vi "ServiceModeTest5.vi"(7 "Erd_ParametricVersion ERD #":T1={"ERD Number"=59, "Data Type"=enum."string"} {"ERD Number" format="%.0x"}, 8 "Error In":errorcluster, 9 "UI GEA Inputs":T5={"Source"=228, "Destination"=37} {"Destination" format="%.0x"; "Source" format="%.0x"}, 10 "MC GEA Inputs":T5={"Source"=228, "Destination"=36} {"Destination" format="%.0x"; "Source" format="%.0x"}, 11 "GEA2 Reference In":refnum<k24>) -> (0 "Error Out":errorcluster, 1 "Report Text":string, 2 "Pass/Fail?":bool, 3 "GEA2 Reference Out":refnum<k24>)   [LabVIEW 2016]
uses:
  Q:/Common/DLLs/GEA3/GeaCommunication.dll
  Common/DLLs/GEA3/GeaCommunication.dll
  Common/LabVIEW GEA2 Toolkit/LabVIEW_GEA2_Toolkit.lvlibp/type defs/Source_Destination.ctl
  Centauro Washer/Product Testcode/Centauro/Valew Common/type defs/LED Status OOB.ctl
  Common/LabVIEW GEA2 Toolkit/LabVIEW_GEA2_Toolkit.lvlibp/type defs/ERD Read Data In.ctl
  Common/LabVIEW GEA2 Toolkit/LabVIEW_GEA2_Toolkit.lvlibp/type defs/Data Type.ctl
  Common/Type Defs/JL_Buttons.ctl
  Common/LabVIEW GEA2 Toolkit/LabVIEW_GEA2_Toolkit.lvlibp
panel:
  in  "LED Status Cluster":T4
  in  "Board Index":i32
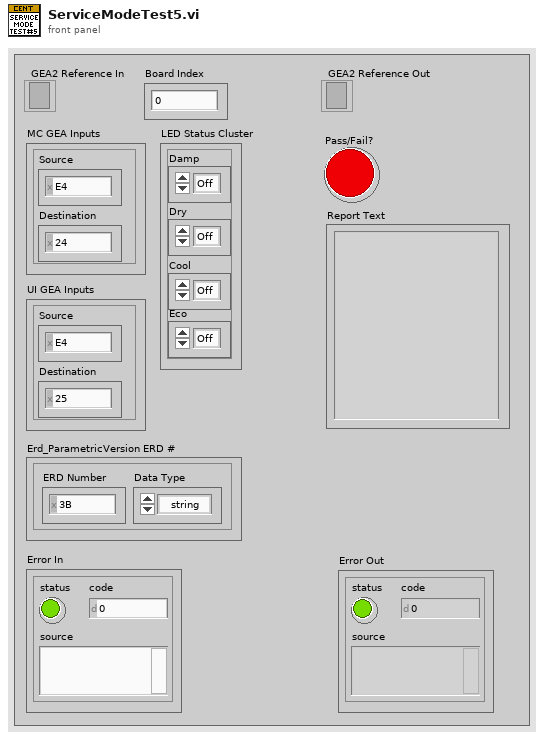
[diagram p1: front panel]
types:
  T1 = typedef "LabVIEW_GEA2_Toolkit.lvlibp/ERD Read Data In.ctl" = cluster{"ERD Number":u16, "Data Type":T2}
  T2 = typedef "LabVIEW_GEA2_Toolkit.lvlibp/Data Type.ctl" = enum16{"string", "boolean", "uint8_t", "uint16_t", "uint32_t", "uint64_t", "int8_t", "int16_t", "int32_t", "int64_t"}
  T3 = typedef "LED Status OOB.ctl" = enum32{"Off", "On", "Blink"}
  T4 = cluster{"Damp":T3, "Dry":T3, "Cool":T3, "Eco":T3}
  T5 = typedef "LabVIEW_GEA2_Toolkit.lvlibp/Source_Destination.ctl" = cluster{"Source":u8, "Destination":u8}
  T6 = typedef "LabVIEW_GEA2_Toolkit.lvlibp/ERD Read Data Out.ctl" = cluster{"ERD Number":u16, "Data":string}
  T7 = typedef "JL_Buttons.ctl" = enum16{"Power", "Start / Pause ", "Temp Option ", "Dryness Level", "Time Option", "Time Increment ", "Time Decrement ", "MyCycle", "eDry ", "Delay", "Extended Tumble", "Control Lock", "Volume/Signal", "Damp Alert / Drum Light", "Unused", "(SW213)", "(SW322)", "Clear / Reset"}
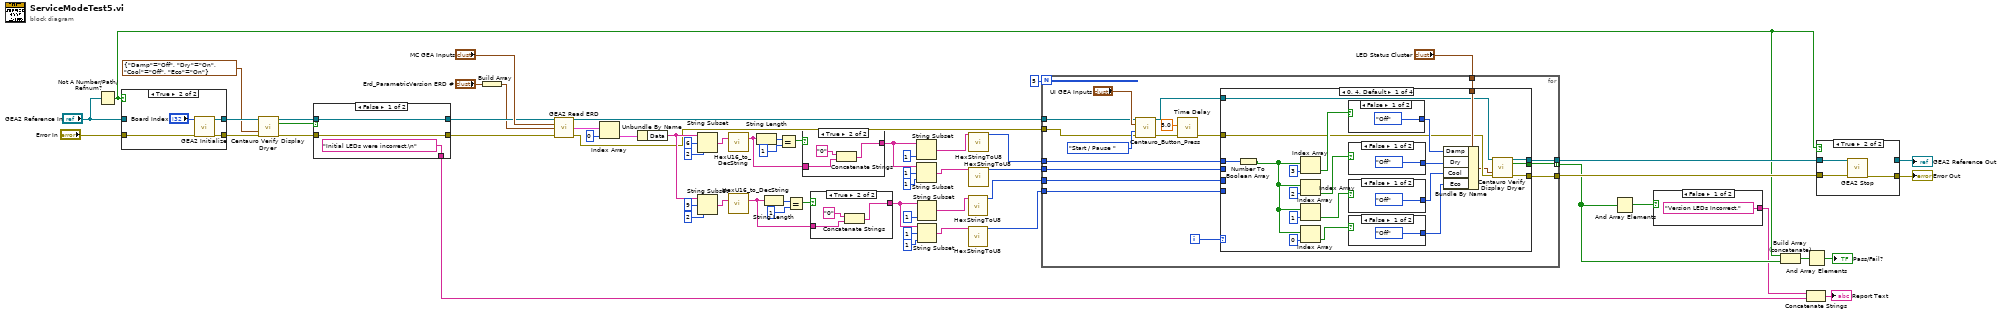
[diagram p0: block diagram]
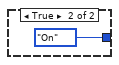
[diagram p5: hidden frame]
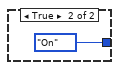
[diagram p6: hidden frame]
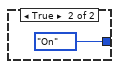
[diagram p7: hidden frame]
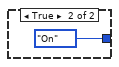
[diagram p8: hidden frame]
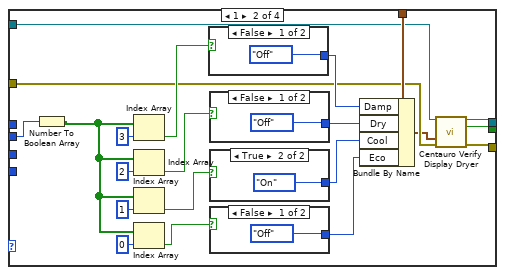
[diagram p9: hidden frame]
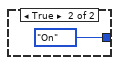
[diagram p10: hidden frame]
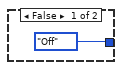
[diagram p11: hidden frame]
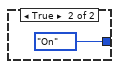
[diagram p12: hidden frame]
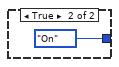
[diagram p13: hidden frame]
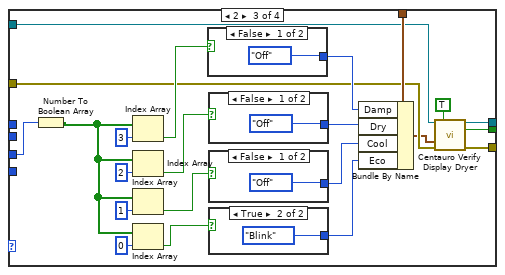
[diagram p14: hidden frame]
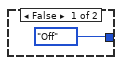
[diagram p15: hidden frame]
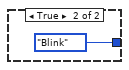
[diagram p16: hidden frame]
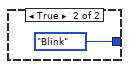
[diagram p17: hidden frame]
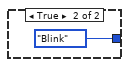
[diagram p18: hidden frame]
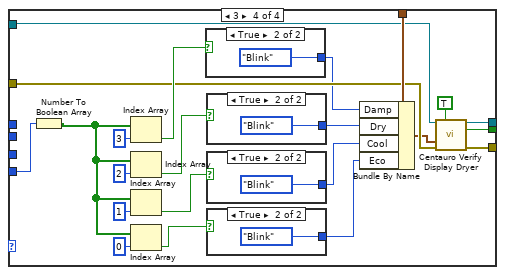
[diagram p19: hidden frame]
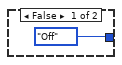
[diagram p20: hidden frame]
diagram:
  n1 = Not A Number/Path/Refnum?(number/path/refnum="GEA2 Reference In") -> (NaN/Path/Refnum?=w31:bool)
  n2 = case shown="True" w31 {
    tunnel: [w64 w69] -> w60
    tunnel: "Error In" -> [w64 w68]
    tunnel: [w65 w67] -> w61
    tunnel: "GEA2 Reference In" -> [w65 _]
    frame False {
    }
    frame True {
      n3 = call "GEA2 Initialize.vi"("Board Index"="Board Index", "error in"=w68) -> ("GEA2 Reference Out"=w67:refnum<k24>, "error out"=w69:errorcluster)  [unwired: 11 in, 1 out]
    }
  }
  n4 = call "Centauro Verify Display Dryer.vi"("GEA2 Reference In"=w61, "Expected LED Status"=T4 {"Damp"=enum."Off", "Dry"=enum."On", "Cool"=enum."Off", "Eco"=enum."On"}, "Error In"=w60) -> ("GEA2 Reference Out"=w59:refnum<k24>, "Pass/Fail?"=w53:bool, "Error Out"=w58:errorcluster)  [unwired: 7 in, 3 out]
  n5 = case shown="False" w53 {
    tunnel: w59 -> [w72 w74]
    tunnel: [w72 w74] -> w43
    tunnel: [w71 w73] -> w42
    tunnel: w58 -> [w71 w73]
    tunnel: ["Initial LEDs were incorrect.\n" _] -> w52
    frame False {
    }
    frame True {
    }
  }
  n6 = Build Array("Erd_ParametricVersion ERD #") -> (w2:T1[])
  n7 = call "GEA2 Read ERD.vi"("GEA2 Reference In"=w43, "GEA Inputs"="MC GEA Inputs", "Read ERD List"=w2, "Error In"=w42) -> ("GEA2 Reference Out"=w41:refnum<k24>, "ERD Data Out"=w56:T6[], "Error Out"=w40:errorcluster)  [unwired: 8 in, 1 out]
  n8 = Index Array(array=w56, index=0) -> (element=w54:T6)
  n9 = Unbundle By Name(w54) -> ("Data"=w45:string)
  n10 = String Subset(string=w45, offset (0)=6, length (rest)=2 ("length (rest)")) -> (substring=w25:string)
  n11 = String Subset(string=w45, offset (0)=9, length (rest)=2 ("length (rest)")) -> (substring=w24:string)
  n12 = call "HexU16_to_DecString.vi"("String"=w25) -> ("decimal integer string"=w20:string)  [unwired: 13 in, 1 out]
  n13 = call "HexU16_to_DecString.vi"("String"=w24) -> ("decimal integer string"=w16:string)  [unwired: 13 in, 1 out]
  n14 = String Length(string=w20) -> (length=w23:i32)
  n15 = String Length(string=w16) -> (length=w19:i32)
  n16 = Equal?(x=w23, y=1) -> (x = y?=w21:bool)
  n17 = Equal?(x=w19, y=1) -> (x = y?=w17:bool)
  n18 = case shown="True" w21 {
    tunnel: w20 -> [w75 w77]
    tunnel: [w75 w76] -> w14
    frame False {
    }
    frame True {
      n19 = Concatenate Strings("0" ("string"), w77) -> (w76:string)
    }
  }
  n20 = case shown="True" w17 {
    tunnel: w16 -> [w79 w81]
    tunnel: [w79 w80] -> w6
    frame False {
    }
    frame True {
      n21 = Concatenate Strings("0" ("string"), w81) -> (w80:string)
    }
  }
  n22 = String Subset(string=w14, length (rest)=1 ("length (rest)")) -> (substring=w11:string)  [unwired: 1 in]
  n23 = String Subset(string=w14, offset (0)=1, length (rest)=1 ("length (rest)")) -> (substring=w10:string)
  n24 = String Subset(string=w6, length (rest)=1 ("length (rest)")) -> (substring=w5:string)  [unwired: 1 in]
  n25 = String Subset(string=w6, offset (0)=1, length (rest)=1 ("length (rest)")) -> (substring=w4:string)
  n26 = call "HexStringToU8.vi"("Input String"=w5) -> ("Number Out"=w37:u8)  [unwired: 14 in]
  n27 = call "HexStringToU8.vi"("Input String"=w4) -> ("Number Out"=w36:u8)  [unwired: 14 in]
  n28 = call "HexStringToU8.vi"("Input String"=w11) -> ("Number Out"=w39:u8)  [unwired: 14 in]
  n29 = call "HexStringToU8.vi"("Input String"=w10) -> ("Number Out"=w38:u8)  [unwired: 14 in]
  n30 = for {
    N: 5 -> [_]
    tunnel: w41 -> [w96]
    tunnel: w40 -> [w95]
    tunnel: w39 -> [w94]
    tunnel: w38 -> [w93]
    tunnel: w37 -> [w92]
    tunnel: w36 -> [w91]
    tunnel: "LED Status Cluster" -> [w90]
    tunnel: [w88] -> w32 mode=indexing
    tunnel: [w87] -> w34
    tunnel: [w86] -> w33
    i -> [w99]
    n31 = call "Centauro_Button_Press.vi"("GEA2 Reference In"=w96, "GEA Inputs"="UI GEA Inputs", "Button"=JL_Buttons."Start / Pause ", "Error In"=w95) -> ("GEA2 Reference Out"=w89:refnum<k24>, "Error Out"=w84:errorcluster)  [unwired: 10 in]
    n32 = call "Time Delay"("error in (no error)"=w84, "Delay Time (s)"=5.0) -> ("error out"=w83:errorcluster)  [unwired: 9 in]
    n33 = case shown="0, 4, Default" w99 {
      tunnel: w94 -> [w120 _ _ _]
      tunnel: w93 -> [_ w140 _ _]
      tunnel: w92 -> [_ _ w170 _]
      tunnel: w91 -> [_ _ _ w200]
      tunnel: w90 -> [w110 w139 w169 w199]
      tunnel: w89 -> [w105 w134 w164 w198]
      tunnel: w83 -> [w104 w133 w163 w197]
      tunnel: [w103 w132 w162 w196] -> w88
      tunnel: [w102 w131 w161 w195] -> w87
      tunnel: [w101 w130 w160 w194] -> w86
      frame 0, 4, Default {
        n34 = Number To Boolean Array(number=w120) -> (Boolean array=w115:bool[])
        n35 = Index Array(array=w115, index=3) -> (element=w114:bool)
        n36 = Index Array(array=w115, index=2) -> (element=w113:bool)
        n37 = Index Array(array=w115, index=1) -> (element=w112:bool)
        n38 = Index Array(array=w115, index=0) -> (element=w111:bool)
        n39 = case shown="False" w114 {
          tunnel: [LED_Status_OOB."Off" ("Damp") LED_Status_OOB."On" ("Damp")] -> w109
          frame False {
          }
          frame True {
          }
        }
        n40 = case shown="False" w113 {
          tunnel: [LED_Status_OOB."Off" ("Damp") LED_Status_OOB."On" ("Damp")] -> w108
          frame False {
          }
          frame True {
          }
        }
        n41 = case shown="False" w112 {
          tunnel: [LED_Status_OOB."Off" ("Damp") LED_Status_OOB."On" ("Damp")] -> w107
          frame False {
          }
          frame True {
          }
        }
        n42 = case shown="False" w111 {
          tunnel: [LED_Status_OOB."Off" ("Damp") LED_Status_OOB."On" ("Damp")] -> w106
          frame False {
          }
          frame True {
          }
        }
        n43 = Bundle By Name(cluster=w110, "Damp"=w109, "Dry"=w108, "Cool"=w107, "Eco"=w106) -> (w100:T4)
        n44 = call "Centauro Verify Display Dryer.vi"("GEA2 Reference In"=w105, "Expected LED Status"=w100, "Error In"=w104) -> ("GEA2 Reference Out"=w102:refnum<k24>, "Pass/Fail?"=w103:bool, "Error Out"=w101:errorcluster)  [unwired: 7 in, 3 out]
      }
      frame 1 {
        n45 = Number To Boolean Array(number=w140) -> (Boolean array=w145:bool[])
        n46 = Index Array(array=w145, index=3) -> (element=w144:bool)
        n47 = Index Array(array=w145, index=2) -> (element=w143:bool)
        n48 = Index Array(array=w145, index=1) -> (element=w142:bool)
        n49 = Index Array(array=w145, index=0) -> (element=w141:bool)
        n50 = case shown="False" w144 {
          tunnel: [LED_Status_OOB."Off" ("Damp") LED_Status_OOB."On" ("Damp")] -> w138
          frame False {
          }
          frame True {
          }
        }
        n51 = case shown="False" w143 {
          tunnel: [LED_Status_OOB."Off" ("Damp") LED_Status_OOB."On" ("Damp")] -> w137
          frame False {
          }
          frame True {
          }
        }
        n52 = case shown="True" w142 {
          tunnel: [LED_Status_OOB."Off" ("Damp") LED_Status_OOB."On" ("Damp")] -> w136
          frame False {
          }
          frame True {
          }
        }
        n53 = case shown="False" w141 {
          tunnel: [LED_Status_OOB."Off" ("Damp") LED_Status_OOB."On" ("Damp")] -> w135
          frame False {
          }
          frame True {
          }
        }
        n54 = Bundle By Name(cluster=w139, "Damp"=w138, "Dry"=w137, "Cool"=w136, "Eco"=w135) -> (w129:T4)
        n55 = call "Centauro Verify Display Dryer.vi"("GEA2 Reference In"=w134, "Expected LED Status"=w129, "Error In"=w133) -> ("GEA2 Reference Out"=w131:refnum<k24>, "Pass/Fail?"=w132:bool, "Error Out"=w130:errorcluster)  [unwired: 7 in, 3 out]
      }
      frame 2 {
        n56 = Number To Boolean Array(number=w170) -> (Boolean array=w175:bool[])
        n57 = Index Array(array=w175, index=3) -> (element=w174:bool)
        n58 = Index Array(array=w175, index=2) -> (element=w173:bool)
        n59 = Index Array(array=w175, index=1) -> (element=w172:bool)
        n60 = Index Array(array=w175, index=0) -> (element=w171:bool)
        n61 = case shown="False" w174 {
          tunnel: [LED_Status_OOB."Off" ("Damp") LED_Status_OOB."Blink" ("Damp")] -> w168
          frame False {
          }
          frame True {
          }
        }
        n62 = case shown="False" w173 {
          tunnel: [LED_Status_OOB."Off" ("Damp") LED_Status_OOB."Blink" ("Damp")] -> w167
          frame False {
          }
          frame True {
          }
        }
        n63 = case shown="False" w172 {
          tunnel: [LED_Status_OOB."Off" ("Damp") LED_Status_OOB."Blink" ("Damp")] -> w166
          frame False {
          }
          frame True {
          }
        }
        n64 = case shown="True" w171 {
          tunnel: [LED_Status_OOB."Off" ("Damp") LED_Status_OOB."Blink" ("Damp")] -> w165
          frame False {
          }
          frame True {
          }
        }
        n65 = Bundle By Name(cluster=w169, "Damp"=w168, "Dry"=w167, "Cool"=w166, "Eco"=w165) -> (w158:T4)
        n66 = call "Centauro Verify Display Dryer.vi"("GEA2 Reference In"=w164, "Service Mode?"=TRUE, "Expected LED Status"=w158, "Error In"=w163) -> ("GEA2 Reference Out"=w161:refnum<k24>, "Pass/Fail?"=w162:bool, "Error Out"=w160:errorcluster)  [unwired: 6 in, 3 out]
      }
      frame 3 {
        n67 = Number To Boolean Array(number=w200) -> (Boolean array=w205:bool[])
        n68 = Index Array(array=w205, index=3) -> (element=w204:bool)
        n69 = Index Array(array=w205, index=2) -> (element=w203:bool)
        n70 = Index Array(array=w205, index=1) -> (element=w202:bool)
        n71 = Index Array(array=w205, index=0) -> (element=w201:bool)
        n72 = case shown="True" w204 {
          tunnel: [LED_Status_OOB."Off" ("Damp") LED_Status_OOB."Blink" ("Damp")] -> w193
          frame False {
          }
          frame True {
          }
        }
        n73 = case shown="True" w203 {
          tunnel: [LED_Status_OOB."Off" ("Damp") LED_Status_OOB."Blink" ("Damp")] -> w192
          frame False {
          }
          frame True {
          }
        }
        n74 = case shown="True" w202 {
          tunnel: [LED_Status_OOB."Off" ("Damp") LED_Status_OOB."Blink" ("Damp")] -> w191
          frame False {
          }
          frame True {
          }
        }
        n75 = case shown="True" w201 {
          tunnel: [LED_Status_OOB."Off" ("Damp") LED_Status_OOB."Blink" ("Damp")] -> w190
          frame False {
          }
          frame True {
          }
        }
        n76 = Bundle By Name(cluster=w199, "Damp"=w193, "Dry"=w192, "Cool"=w191, "Eco"=w190) -> (w188:T4)
        n77 = call "Centauro Verify Display Dryer.vi"("GEA2 Reference In"=w198, "Service Mode?"=TRUE, "Expected LED Status"=w188, "Error In"=w197) -> ("GEA2 Reference Out"=w195:refnum<k24>, "Pass/Fail?"=w196:bool, "Error Out"=w194:errorcluster)  [unwired: 6 in, 3 out]
      }
    }
  }
  n78 = And Array Elements(Boolean array=w32) -> (logical AND=w28:bool)
  n79 = case shown="False" w28 {
    tunnel: ["Version LEDs Incorrect." _] -> w26
    frame False {
    }
    frame True {
    }
  }
  n80 = Build Array (concatenate)(w31, w32) -> (w30:bool[])
  n81 = Concatenate Strings(w26, w52) -> (→"Report Text":string)
  n82 = And Array Elements(Boolean array=w30) -> (logical AND=→"Pass/Fail?":bool)
  n83 = case shown="True" w31 {
    tunnel: [w219 w223] -> w50
    tunnel: w34 -> [w220 w222]
    tunnel: w33 -> [w219 w221]
    tunnel: [w220 _] -> w27
    frame False {
    }
    frame True {
      n84 = call "GEA2 Stop.vi"("GEA2 Reference In"=w222, "Error In"=w221) -> ("Error Out"=w223:errorcluster)  [unwired: 13 in]
    }
  }
  "GEA2 Reference Out" <- w27
  "Error Out" <- w50
